vi "Guage.vi"() -> ()   [LabVIEW 2013]
panel:
  out "Waveform Chart":dbl(graph)
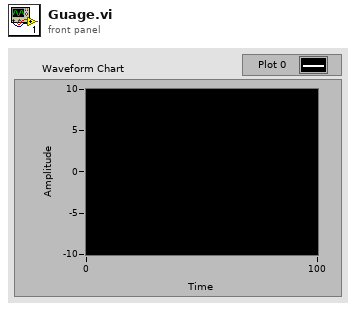
[diagram p1: front panel]
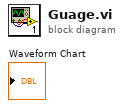
[diagram p0: block diagram]
diagram:
